vi "getNumBuckets.vi"(8 "error in (no error)":errorcluster, 11 "HashMap in":refnum<class "HashMap.lvclass">) -> (0 "error out":errorcluster, 2 "NumBuckets":i32, 3 "HashMap out":refnum<class "HashMap.lvclass">)   [LabVIEW 2017, in "HashMap.lvclass"]
uses:
  <userlib>/836-Library/Data_Structures/HashMap/HashMap.lvclass
  <userlib>/836-Library/Data_Structures/HashMap/HashMap.lvclass/HashMap.ctl
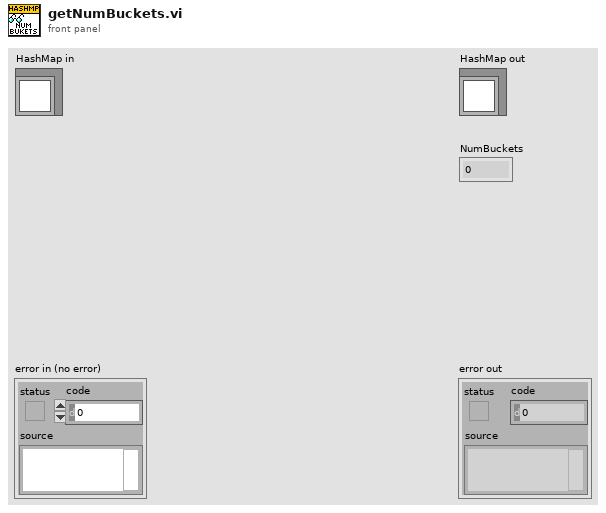
[diagram p1: front panel]
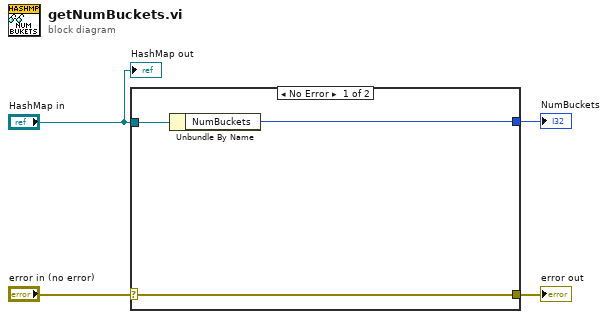
[diagram p0: block diagram]
diagram:
  n1 = case shown="No Error" "error in (no error)" {
    selector: "error in (no error)" -> [w7 w8]
    tunnel: [w7 w8] -> w3
    tunnel: "HashMap in" -> [w6 _]
    tunnel: [w5 _] -> w2
    frame No Error {
      n2 = Unbundle By Name(w6) -> ("NumBuckets"=w5:i32)
    }
    frame Error {
    }
  }
  "error out" <- w3
  "NumBuckets" <- w2
  "HashMap out" <- "HashMap in"
